vi "Actor Core.vi"(8 "error in":errorcluster, 11 "Laser_Oxxius in":refnum<class "Laser_Oxxius.lvclass">) -> (0 "error out":errorcluster, 3 "Actor out":refnum<class "Actor.lvclass">)   [LabVIEW 2020, in "Laser_Oxxius.lvlib" / "Laser_Oxxius.lvclass"]
doc: "(<B>Filename</B>: Actor Framework.lvlib:Actor.lvclass:Actor Core.vi)\n\nReceives messages to the actor, reacts to them, and initiates any error handling that may shut the actor down.\n\nDescendant classes may override this VI to append parallel tasks for the actor to complete while it handles messages. Overrides use the Call Parent Class Method node."
uses:
  Laser_Oxxius.lvclass
  C:/Program Files/National Instruments/LabVIEW 2020/vi.lib/ActorFramework/Actor/Actor.lvclass
  <vilib>/ActorFramework/Actor/Actor.lvclass
  Laser Oxxius Controller/Laser Oxxius Controller.lvclass
  Laser_Oxxius.lvclass/Laser_Oxxius.ctl
  Laser Oxxius Controller Messages/Update UI Msg/Update UI Msg.lvclass/Update UI Msg.ctl
  <vilib>/ActorFramework/Message Enqueuer/Message Enqueuer.lvclass/Message Enqueuer.ctl
  <vilib>/ActorFramework/Message Enqueuer/Enqueue.vi
  Laser Oxxius Controller Messages/Update UI Msg/Update UI Msg.lvclass
  C:/Program Files/National Instruments/LabVIEW 2020/vi.lib/ActorFramework/Message/Message.lvclass
  <vilib>/ActorFramework/Message Priority Queue/Priority Enqueue.vi
  HAL Layer/Component/Laser/Laser/Laser.lvclass
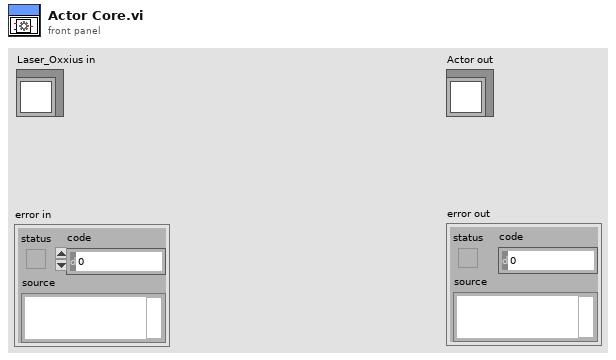
[diagram p1: front panel]
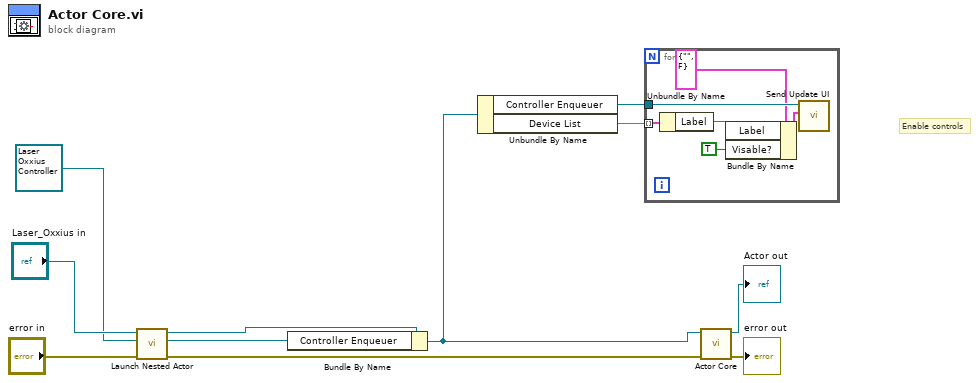
[diagram p0: block diagram]
diagram:
  # "Enable controls"
  n1 = call <vilib>:"Launch Nested Actor.vi"("error in (no error)"="error in", "Nested Actor"=refnum<class "Laser Oxxius Controller.lvclass"> refnum ("Laser_Oxxius.lvlib:Laser Oxxius Controller.lvlib:Laser Oxxius Controller.lvclass"), "Caller Actor in"="Laser_Oxxius in") -> ("error out"=w7:errorcluster, "Nested Actor's Enqueuer"=w9:refnum<class "Message Enqueuer.lvclass">, "Caller Actor out"=w5:refnum<class "Laser_Oxxius.lvclass">)  [unwired: 6 in]
  n2 = Bundle By Name(cluster=w5, "Controller Enqueuer"=w9) -> (w3:refnum<class "Laser_Oxxius.lvclass">)
  n3 = Unbundle By Name(w3) -> ("Controller Enqueuer"=w1:refnum<class "Message Enqueuer.lvclass">, "Device List"=w2:map{string, refnum<k24>})
  n4 = for {
    tunnel: w2 -> [w17] mode=indexing
    tunnel: w1 -> [w16]
    n5 = Unbundle By Name(w17) -> ("Label"=w13:string)
    n6 = Bundle By Name(cluster=cluster{"Label":string, "Visable?":bool} {"Label"="", "Visable?"=FALSE} ("event data"), "Label"=w13, "Visable?"=TRUE) -> (w14:cluster{"Label":string, "Visable?":bool})
    n7 = call "Send Update UI.vi"("event data"=w14, "Message Enqueuer"=w16) -> ()  [unwired: 8 in, 2 out]
  }
  n8 = call-parent "Actor Core.vi"("error in"=w7, "Actor in"=w3) -> ("error out"=→"error out":errorcluster, "Actor out"=→"Actor out":refnum<class "Actor.lvclass">)  [unwired: 8 in]
